vi "TimingFunctions_convertLvToJavaTimestamp.vi"(1 "TimeStamp (LV)":timestamp format="%^<%H:%M:%S%3u %p\n%d/%m/%Y>T") -> (15 "TimeStamp (Java)":u64, 16 "TimeStampString (Java)":string)   [LabVIEW 2016]
doc: "Konvertiert einen LV Timestamp in einen Timestamp startend am 1.1.1970, in 1/1000s Schritten, U64\n\n15.05.14 / sige"
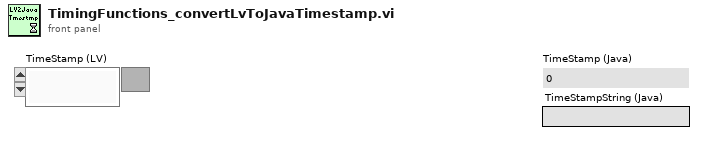
[diagram p1: front panel]
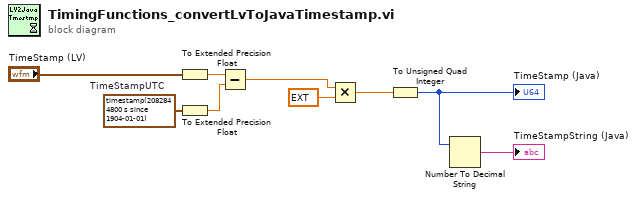
[diagram p0: block diagram]
diagram:
  w4 = timestamp(2082844800 s since 1904-01-01)  # TimeStampUTC
  n1 = To Extended Precision Float(1:"TimeStamp (LV)") -> (0:w8:ext)
  n2 = To Extended Precision Float(1:w4) -> (0:w5:ext)
  n3 = Subtract(x=w8, y=w5) -> (x-y=w6:ext)
  n4 = Multiply(x=w6, y=ext 1000.0) -> (x*y=w3:ext)
  n5 = To Unsigned Quad Integer(1:w3) -> (0:w2:u64)
  "TimeStamp (Java)" <- w2
  n6 = Number To Decimal String(number=w2) -> (decimal integer string=→"TimeStampString (Java)":string)  [unwired: 1 in]
